vi "Get Directory Listing.vi"(8 "error in (no error)":errorcluster, 10 "RemoteDirectory":string, 11 "FTP in":refnum<class "FTP.lvclass">) -> (0 "error out":errorcluster, 2 "Dir-File Info Array":T1[](array[typedef]), 3 "FTP out":refnum<class "FTP.lvclass">)   [LabVIEW 2020, in "FTP.lvlib" / "FTP.lvclass"]
doc: "Gets a directory listing of the remote server's directory. The directory listing is returned by an array of clusters. The cluster contains information about the folders and files contained within the remote server's directory."
uses:
  FTP.lvclass
  controls/Dir-File Info.ctl
  controls/Dir-File Type.ctl
  FTP.lvclass/FTP.ctl
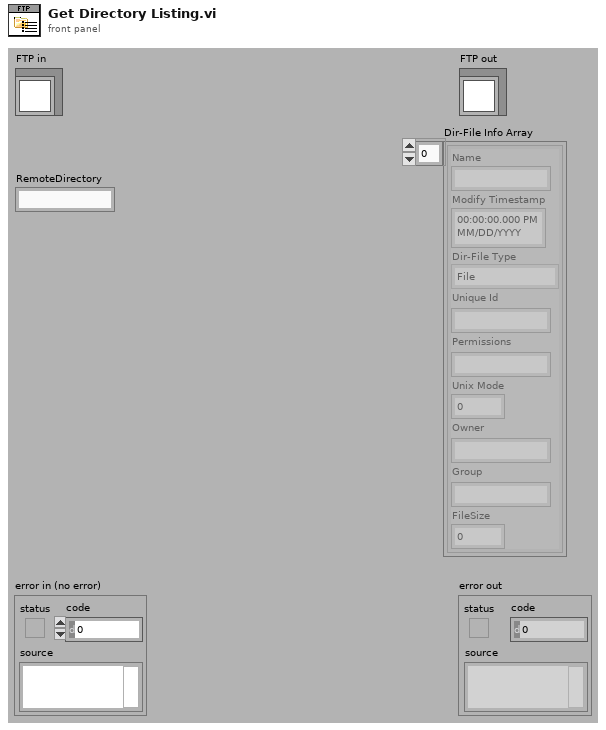
[diagram p1: front panel]
types:
  T1 = typedef "FTP.lvlib/FTP.lvclass/Dir-File Info.ctl" = cluster{"Name":string, "Modify Timestamp":timestamp, "Dir-File Type":T2, "Unique Id":string, "Permissions":string, "Unix Mode":u16, "Owner":string, "Group":string, "FileSize":i64}
  T2 = typedef "FTP.lvlib/FTP.lvclass/Dir-File Type.ctl" = enum16{"File", "Listed Directory", "Parent Directory", "Directory", "Unknown"}
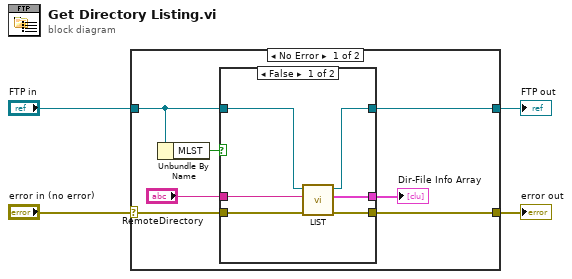
[diagram p0: block diagram]
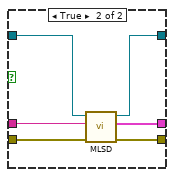
[diagram p2: hidden frame]
diagram:
  n1 = case shown="No Error" "error in (no error)" {
    selector: "error in (no error)" -> [w11 w25]
    tunnel: [w8 w25] -> w3
    tunnel: [w7 w24] -> w1
    tunnel: "FTP in" -> [w6 w24]
    frame No Error {
      n2 = Unbundle By Name(w6) -> ("MLST"=w5:bool)
      n3 = case shown="False" w5 {
        tunnel: w11 -> [w17 w23]
        tunnel: "RemoteDirectory" -> [w13 w22]
        tunnel: [w12 w21] -> w9
        tunnel: [w16 w20] -> w8
        tunnel: w6 -> [w15 w19]
        tunnel: [w14 w18] -> w7
        frame False {
          n4 = call "LIST.vi"("error in (no error)"=w17, "Remote File"=w13, "FTP in"=w15) -> ("error out"=w16:errorcluster, "Dir-File Info Array"=w12:T1[], "FTP out"=w14:refnum<class "FTP.lvclass">)  [unwired: 6 in]
        }
        frame True {
          n5 = call "MLSD.vi"("error in (no error)"=w23, "RemoteDirectory"=w22, "FTP in"=w19) -> ("error out"=w20:errorcluster, "Dir-File Info Array"=w21:T1[], "FTP out"=w18:refnum<class "FTP.lvclass">)  [unwired: 6 in]
        }
      }
      "Dir-File Info Array" <- w9
    }
    frame Error {
    }
  }
  "error out" <- w3
  "FTP out" <- w1
